vi "global_read.vi"(10 "Boolean":bool) -> ()   [LabVIEW 2011]
uses:
  <vilib>/Utility/file.llb/Read From Spreadsheet File (string).vi
  Robot Global Data.vi
panel:
  in  "format (%.3f) 2":string="%.3f"
  in  "delimiter (\\t) 2":string=","
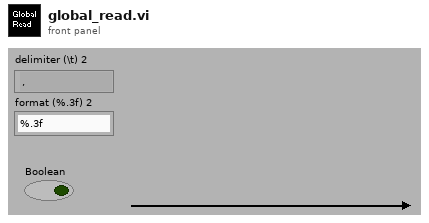
[diagram p1: front panel]
types:
  T1 = cluster{"all rows[0]":string, "all rows[1]":string}
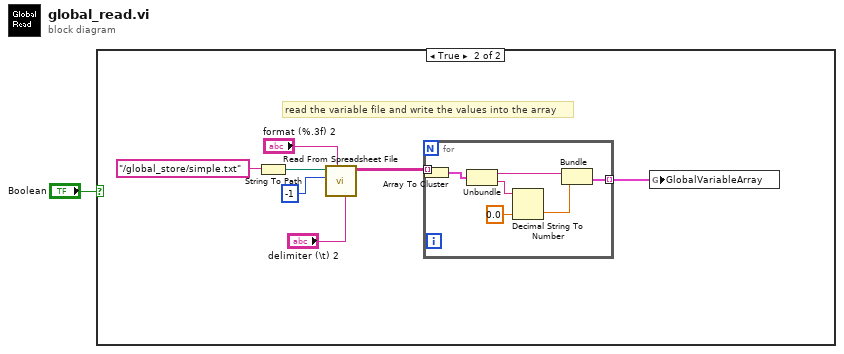
[diagram p0: block diagram]
diagram:
  n1 = case shown="True" "Boolean" {
    frame False {
    }
    frame True {
      # "read the variable file and write the values into the array"
      n2 = String To Path(string="/global_store/simple.txt") -> (path=w3:path)
      n3 = call-poly <vilib>:"Read From Spreadsheet File.vi"("delimiter (\\t)"="delimiter (\\t) 2", "format (%s)"="format (%.3f) 2", "number of rows (all:-1)"=-1, "file path (dialog if empty)"=w3) -> ("all rows"=w5:string[][])  [unwired: 1 in, 6 out]
      n4 = for {
        tunnel: w5 -> [w15] mode=indexing
        tunnel: [w9] -> w4 mode=indexing
        n5 = Array To Cluster(array=w15) -> (cluster=w14:T1)
        n6 = Unbundle(w14) -> ("all rows[0]"=w13:string, "all rows[1]"=w12:string)
        n7 = Decimal String To Number(string=w12, default (0L)=0.0 ("default (0 I32)")) -> (number=w11:dbl)  [unwired: 2 out]
        n8 = Bundle("all rows[0]"=w13, w11) -> (w9:cluster{"all rows[0]":string, dbl})  [unwired: 1 out]
      }
      n9 = global write "Robot Global Data.vi" "GlobalVariableArray"(w4) -> ()
    }
  }
